vi "Version_4.9_8_on-chip_valves_for25ulSyringe_withModfied_Plunging.vi"() -> ()   [LabVIEW 2020] (continued)
                            n6063 = local write "Volume being Injected \nin this process"(0.0 ("Volume being Injected \nin this process")) -> ()
                          }
                        }
                      }
                      frame #5 {
                        n6064 = while {
                          stop <- w6523 stop-if-true
                          # "Re-introduce Sample into Column-2, Elute column-2 and Divert the sample onto Grid"
                          n6065 = local read "Start the Process"() -> (w6522:bool)
                          n6066 = case shown="True" w6522 {
                            frame False {
                            }
                            frame True {
                              n6067 = stacked-sequence {
                                frame #0 {
                                # "Reinitialize the pump"
                                n6068 = local read "VISA Refnum in\nfor Pump"() -> (w6525:refnum<visa-resource-name>)
                                n6069 = call "Initializer (SubVI).vi"("VISA Refnum in"=w6525) -> ()  [unwired: 11 in]
                                n6070 = local write "Re-SEC"(FALSE ("Re-SEC")) -> ()
                                }
                                frame #1 {
                                # "If Yes, this code will clean the column-2 with buffer-C prior to re-introducing the sample"
                                n6071 = local read "Wash column-2 Prior \nto re-introducing \nsample"() -> (w6526:bool)
                                n6072 = case shown="True" w6526 {
                                frame False {
                                }
                                frame True {
                                n6073 = stacked-sequence {
                                frame #0 {
                                n6074 = local read "VISA Refnum in\nfor Pump"() -> (w6528:refnum<visa-resource-name>)
                                n6075 = local read "Port for \nC2-Elution"() -> (w6527:string)
                                n6076 = call "PortChanger (SubVI).vi"("Port Number"=w6527, "VISA Refnum in"=w6528) -> ()  [unwired: 10 in]
                                }
                                frame #1 {
                                n6077 = local read "Stopper that ends \nthe main loops"() -> (w6529:bool)
                                n6078 = local read "VISA Refnum in\nfor Pump"() -> (w6530:refnum<visa-resource-name>)
                                n6079 = case shown="True" w6529 {
                                frame False {
                                }
                                frame True {
                                n6080 = local read "VISA Refnum in\nfor Pump"() -> (w6531:refnum<visa-resource-name>)
                                n6081 = call "HardStopCurrentProcess (SubVI).vi"("VISA Refnum in"=w6531) -> ()  [unwired: 11 in]
                                }
                                }
                                n6082 = call "ProcessCompletionWaiter (SubVI).vi"("VISA Refnum in"=w6530) -> ()  [unwired: 11 in]
                                }
                                frame #2 {
                                n6083 = local read "Buffer-B Pumping\nResolution"() -> (w6534:T2)
                                n6084 = local read "VISA Refnum in\nfor Pump"() -> (w6536:refnum<visa-resource-name>)
                                n6085 = local read "Buffer-C2 \nWash Volume\nPrior to re-introducing \nSample"() -> (w6533:dbl)
                                n6086 = local read "Volume of Syringe"() -> (w6535:dbl)
                                n6087 = call "RPickUp(SubVI).vi"("Volume to be picked up"=w6533, "Volume of Syringe"=w6535, "Resolution of PickUP"=w6534, "PickUp Flow Rate (ul/min)"=150.0, "VISA Refnum in"=w6536) -> ()  [unwired: 6 in, 1 out]
                                }
                                frame #3 {
                                n6088 = local read "Stopper that ends \nthe main loops"() -> (w6537:bool)
                                n6089 = local read "VISA Refnum in\nfor Pump"() -> (w6538:refnum<visa-resource-name>)
                                n6090 = case shown="True" w6537 {
                                frame False {
                                }
                                frame True {
                                n6091 = local read "VISA Refnum in\nfor Pump"() -> (w6539:refnum<visa-resource-name>)
                                n6092 = call "HardStopCurrentProcess (SubVI).vi"("VISA Refnum in"=w6539) -> ()  [unwired: 11 in]
                                }
                                }
                                n6093 = call "ProcessCompletionWaiter (SubVI).vi"("VISA Refnum in"=w6538) -> ()  [unwired: 11 in]
                                }
                                frame #4 {
                                n6094 = local read "VISA Refnum in\nfor Pump"() -> (w6541:refnum<visa-resource-name>)
                                n6095 = call "PortChanger (SubVI).vi"("Port Number"="10", "VISA Refnum in"=w6541) -> ()  [unwired: 10 in]
                                }
                                frame #5 {
                                n6096 = local read "Stopper that ends \nthe main loops"() -> (w6542:bool)
                                n6097 = local read "VISA Refnum in\nfor Pump"() -> (w6543:refnum<visa-resource-name>)
                                n6098 = case shown="True" w6542 {
                                frame False {
                                }
                                frame True {
                                n6099 = local read "VISA Refnum in\nfor Pump"() -> (w6544:refnum<visa-resource-name>)
                                n6100 = call "HardStopCurrentProcess (SubVI).vi"("VISA Refnum in"=w6544) -> ()  [unwired: 11 in]
                                }
                                }
                                n6101 = call "ProcessCompletionWaiter (SubVI).vi"("VISA Refnum in"=w6543) -> ()  [unwired: 11 in]
                                }
                                frame #6 {
                                n6102 = local read "Buffer-C2 Dispense \nFlow Rate for Washing \nPrior to re-introducing Sample"() -> (w6545:dbl)
                                n6103 = local read "VISA Refnum in\nfor Pump"() -> (w6549:refnum<visa-resource-name>)
                                n6104 = local read "Volume of Syringe"() -> (w6547:dbl)
                                n6105 = call "GoToAbsolutePosition(SubVI).vi"("Absolute Volume Position in Syringe (in ul)"=0.0, "Volume of Syringe"=w6547, "Resolution of Pumping"=T2."Standard Pumping", "Flow Rate (ul/min)"=w6545, "VISA Refnum in"=w6549) -> ()  [unwired: 6 in, 1 out]
                                }
                                frame #7 {
                                n6106 = local read "Stopper that ends \nthe main loops"() -> (w6550:bool)
                                n6107 = local read "VISA Refnum in\nfor Pump"() -> (w6551:refnum<visa-resource-name>)
                                n6108 = case shown="True" w6550 {
                                frame False {
                                }
                                frame True {
                                n6109 = local read "VISA Refnum in\nfor Pump"() -> (w6552:refnum<visa-resource-name>)
                                n6110 = call "HardStopCurrentProcess (SubVI).vi"("VISA Refnum in"=w6552) -> ()  [unwired: 11 in]
                                }
                                }
                                n6111 = call "ProcessCompletionWaiter (SubVI).vi"("VISA Refnum in"=w6551) -> ()  [unwired: 11 in]
                                }
                                }
                                }
                                }
                                }
                                frame #2 {
                                # "Switch to Port-7"
                                # "Port-7 of pump is connected to Buffer-B"
                                n6112 = local write "Washing Column-2"(FALSE ("Washing Column-2")) -> ()
                                n6113 = local read "VISA Refnum in\nfor Pump"() -> (w6559:refnum<visa-resource-name>)
                                n6114 = local read "Port for \nB-Elution"() -> (w6557:string)
                                n6115 = local write "Affinity Elution On"(TRUE ("Affinity Elution On")) -> ()
                                n6116 = call "PortChanger (SubVI).vi"("Port Number"=w6557, "VISA Refnum in"=w6559) -> ()  [unwired: 10 in]
                                n6117 = local write "Elution of Column-1"(TRUE ("Elution of Column-1")) -> ()
                                n6118 = local write "Clean the \nBuffer-B tubing"(FALSE ("Clean the \nBuffer-B tubing")) -> ()
                                n6119 = local write "Divert Sample \ninto Column-2"(TRUE ("Divert Sample \ninto Column-2")) -> ()
                                }
                                frame #3 {
                                n6120 = local read "VISA Refnum in\nfor Pump"() -> (w6560:refnum<visa-resource-name>)
                                n6121 = call "ProcessCompletionWaiter (SubVI).vi"("VISA Refnum in"=w6560) -> ()  [unwired: 11 in]
                                }
                                frame #4 {
                                # "If Yes, it will clean the elution buffer from port-5 tubing a bit more"
                                n6122 = local read "Clean the \nBuffer-B tubing"() -> (w6561:bool)
                                n6123 = case shown="True" w6561 {
                                frame False {
                                n6124 = stacked-sequence {
                                frame #0 {
                                n6125 = local read "Buffer-B Pumping\nResolution"() -> (w6564:T2)
                                n6126 = local read "VISA Refnum in\nfor Pump"() -> (w6566:refnum<visa-resource-name>)
                                n6127 = local read "V-S"() -> (w6563:dbl)
                                n6128 = local read "Volume of Syringe"() -> (w6565:dbl)
                                n6129 = call "RPickUp(SubVI).vi"("Volume to be picked up"=w6563, "Volume of Syringe"=w6565, "Resolution of PickUP"=w6564, "PickUp Flow Rate (ul/min)"=150.0, "VISA Refnum in"=w6566) -> ()  [unwired: 6 in, 1 out]
                                }
                                frame #1 {
                                n6130 = local read "Stopper that ends \nthe main loops"() -> (w6567:bool)
                                n6131 = local read "VISA Refnum in\nfor Pump"() -> (w6568:refnum<visa-resource-name>)
                                n6132 = case shown="True" w6567 {
                                frame False {
                                }
                                frame True {
                                n6133 = local read "VISA Refnum in\nfor Pump"() -> (w6569:refnum<visa-resource-name>)
                                n6134 = call "HardStopCurrentProcess (SubVI).vi"("VISA Refnum in"=w6569) -> ()  [unwired: 11 in]
                                }
                                }
                                n6135 = call "ProcessCompletionWaiter (SubVI).vi"("VISA Refnum in"=w6568) -> ()  [unwired: 11 in]
                                }
                                frame #2 {
                                n6136 = local read "VISA Refnum in\nfor Pump"() -> (w6571:refnum<visa-resource-name>)
                                n6137 = call "PortChanger (SubVI).vi"("Port Number"="1", "VISA Refnum in"=w6571) -> ()  [unwired: 10 in]
                                }
                                frame #3 {
                                n6138 = local read "Stopper that ends \nthe main loops"() -> (w6572:bool)
                                n6139 = local read "VISA Refnum in\nfor Pump"() -> (w6573:refnum<visa-resource-name>)
                                n6140 = case shown="True" w6572 {
                                frame False {
                                }
                                frame True {
                                n6141 = local read "VISA Refnum in\nfor Pump"() -> (w6574:refnum<visa-resource-name>)
                                n6142 = call "HardStopCurrentProcess (SubVI).vi"("VISA Refnum in"=w6574) -> ()  [unwired: 11 in]
                                }
                                }
                                n6143 = call "ProcessCompletionWaiter (SubVI).vi"("VISA Refnum in"=w6573) -> ()  [unwired: 11 in]
                                }
                                frame #4 {
                                n6144 = local read "VISA Refnum in\nfor Pump"() -> (w6579:refnum<visa-resource-name>)
                                n6145 = local read "Volume of Syringe"() -> (w6576:dbl)
                                n6146 = call "GoToAbsolutePosition(SubVI).vi"("Absolute Volume Position in Syringe (in ul)"=0.0, "Volume of Syringe"=w6576, "Resolution of Pumping"=T2."Standard Pumping", "Flow Rate (ul/min)"=150.0, "VISA Refnum in"=w6579) -> ()  [unwired: 6 in, 1 out]
                                }
                                frame #5 {
                                n6147 = local read "Stopper that ends \nthe main loops"() -> (w6580:bool)
                                n6148 = local read "VISA Refnum in\nfor Pump"() -> (w6581:refnum<visa-resource-name>)
                                n6149 = case shown="True" w6580 {
                                frame False {
                                }
                                frame True {
                                n6150 = local read "VISA Refnum in\nfor Pump"() -> (w6582:refnum<visa-resource-name>)
                                n6151 = call "HardStopCurrentProcess (SubVI).vi"("VISA Refnum in"=w6582) -> ()  [unwired: 11 in]
                                }
                                }
                                n6152 = call "ProcessCompletionWaiter (SubVI).vi"("VISA Refnum in"=w6581) -> ()  [unwired: 11 in]
                                }
                                }
                                }
                                frame True {
                                n6153 = for {
                                N: 2 -> [_]
                                n6154 = stacked-sequence {
                                frame #0 {
                                n6155 = local read "Buffer-B Pumping\nResolution"() -> (w6586:T2)
                                n6156 = local read "VISA Refnum in\nfor Pump"() -> (w6588:refnum<visa-resource-name>)
                                n6157 = local read "Apparent Volume\nof Syringe"() -> (w6585:dbl)
                                n6158 = local read "Volume of Syringe"() -> (w6587:dbl)
                                n6159 = call "RPickUp(SubVI).vi"("Volume to be picked up"=w6585, "Volume of Syringe"=w6587, "Resolution of PickUP"=w6586, "PickUp Flow Rate (ul/min)"=150.0, "VISA Refnum in"=w6588) -> ()  [unwired: 6 in, 1 out]
                                }
                                frame #1 {
                                n6160 = local read "Stopper that ends \nthe main loops"() -> (w6589:bool)
                                n6161 = local read "VISA Refnum in\nfor Pump"() -> (w6590:refnum<visa-resource-name>)
                                n6162 = case shown="True" w6589 {
                                frame False {
                                }
                                frame True {
                                n6163 = local read "VISA Refnum in\nfor Pump"() -> (w6591:refnum<visa-resource-name>)
                                n6164 = call "HardStopCurrentProcess (SubVI).vi"("VISA Refnum in"=w6591) -> ()  [unwired: 11 in]
                                }
                                }
                                n6165 = call "ProcessCompletionWaiter (SubVI).vi"("VISA Refnum in"=w6590) -> ()  [unwired: 11 in]
                                }
                                frame #2 {
                                n6166 = local read "VISA Refnum in\nfor Pump"() -> (w6593:refnum<visa-resource-name>)
                                n6167 = call "PortChanger (SubVI).vi"("Port Number"="1", "VISA Refnum in"=w6593) -> ()  [unwired: 10 in]
                                }
                                frame #3 {
                                n6168 = local read "Stopper that ends \nthe main loops"() -> (w6594:bool)
                                n6169 = local read "VISA Refnum in\nfor Pump"() -> (w6595:refnum<visa-resource-name>)
                                n6170 = case shown="True" w6594 {
                                frame False {
                                }
                                frame True {
                                n6171 = local read "VISA Refnum in\nfor Pump"() -> (w6596:refnum<visa-resource-name>)
                                n6172 = call "HardStopCurrentProcess (SubVI).vi"("VISA Refnum in"=w6596) -> ()  [unwired: 11 in]
                                }
                                }
                                n6173 = call "ProcessCompletionWaiter (SubVI).vi"("VISA Refnum in"=w6595) -> ()  [unwired: 11 in]
                                }
                                frame #4 {
                                n6174 = local read "VISA Refnum in\nfor Pump"() -> (w6601:refnum<visa-resource-name>)
                                n6175 = local read "Volume of Syringe"() -> (w6598:dbl)
                                n6176 = call "GoToAbsolutePosition(SubVI).vi"("Absolute Volume Position in Syringe (in ul)"=0.0, "Volume of Syringe"=w6598, "Resolution of Pumping"=T2."Standard Pumping", "Flow Rate (ul/min)"=150.0, "VISA Refnum in"=w6601) -> ()  [unwired: 6 in, 1 out]
                                }
                                frame #5 {
                                n6177 = local read "Stopper that ends \nthe main loops"() -> (w6602:bool)
                                n6178 = local read "VISA Refnum in\nfor Pump"() -> (w6603:refnum<visa-resource-name>)
                                n6179 = case shown="True" w6602 {
                                frame False {
                                }
                                frame True {
                                n6180 = local read "VISA Refnum in\nfor Pump"() -> (w6604:refnum<visa-resource-name>)
                                n6181 = call "HardStopCurrentProcess (SubVI).vi"("VISA Refnum in"=w6604) -> ()  [unwired: 11 in]
                                }
                                }
                                n6182 = call "ProcessCompletionWaiter (SubVI).vi"("VISA Refnum in"=w6603) -> ()  [unwired: 11 in]
                                }
                                }
                                }
                                }
                                }
                                }
                                frame #5 {
                                n6183 = local read "VISA Refnum in\nfor Pump"() -> (w6606:refnum<visa-resource-name>)
                                n6184 = local read "Port for \nB-Elution"() -> (w6605:string)
                                n6185 = call "PortChanger (SubVI).vi"("Port Number"=w6605, "VISA Refnum in"=w6606) -> ()  [unwired: 10 in]
                                }
                                frame #6 {
                                n6186 = local read "VISA Refnum in\nfor Pump"() -> (w6607:refnum<visa-resource-name>)
                                n6187 = call "ProcessCompletionWaiter (SubVI).vi"("VISA Refnum in"=w6607) -> ()  [unwired: 11 in]
                                }
                                frame #7 {
                                n6188 = local read "Buffer-B PickUp \nFlow Rate (ul/min)"() -> (w6610:dbl)
                                n6189 = local read "Buffer-B Pumping\nResolution"() -> (w6609:T2)
                                n6190 = local read "VISA Refnum in\nfor Pump"() -> (w6612:refnum<visa-resource-name>)
                                n6191 = local read "Buffer-B Volume \nto be  Pumped"() -> (w6608:dbl)
                                n6192 = local read "Volume of Syringe"() -> (w6611:dbl)
                                n6193 = call "RPickUp(SubVI).vi"("Volume to be picked up"=w6608, "Volume of Syringe"=w6611, "Resolution of PickUP"=w6609, "PickUp Flow Rate (ul/min)"=w6610, "VISA Refnum in"=w6612) -> ()  [unwired: 6 in, 1 out]
                                }
                                frame #8 {
                                n6194 = local read "Stopper that ends \nthe main loops"() -> (w6613:bool)
                                n6195 = local read "VISA Refnum in\nfor Pump"() -> (w6614:refnum<visa-resource-name>)
                                n6196 = case shown="True" w6613 {
                                frame False {
                                }
                                frame True {
                                n6197 = local read "VISA Refnum in\nfor Pump"() -> (w6615:refnum<visa-resource-name>)
                                n6198 = call "HardStopCurrentProcess (SubVI).vi"("VISA Refnum in"=w6615) -> ()  [unwired: 11 in]
                                }
                                }
                                n6199 = call "ProcessCompletionWaiter (SubVI).vi"("VISA Refnum in"=w6614) -> ()  [unwired: 11 in]
                                }
                                frame #9 {
                                # "Reads the initial Plunger Position for computing the volume dispensed"
                                n6200 = local read "VISA Refnum in\nfor Pump"() -> (w6617:refnum<visa-resource-name>)
                                n6201 = call "AbsolutePlungerPosition (SubVI).vi"("VISA Refnum in"=w6617) -> ("Plunger Position"=w6616:i32)  [unwired: 10 in]
                                n6202 = local write "Initial Plunger Position"(w6616) -> ()
                                }
                                frame #10 {
                                # "Switch to Port-2"
                                # "Port-2 of the pump is conncted to column-1 of chip"
                                n6203 = local read "VISA Refnum in\nfor Pump"() -> (w6619:refnum<visa-resource-name>)
                                n6204 = call "PortChanger (SubVI).vi"("Port Number"="2", "VISA Refnum in"=w6619) -> ()  [unwired: 10 in]
                                }
                                frame #11 {
                                n6205 = local read "Stopper that ends \nthe main loops"() -> (w6620:bool)
                                n6206 = local read "VISA Refnum in\nfor Pump"() -> (w6621:refnum<visa-resource-name>)
                                n6207 = call "ProcessCompletionWaiter (SubVI).vi"("VISA Refnum in"=w6621) -> ()  [unwired: 11 in]
                                n6208 = case shown="True" w6620 {
                                frame False {
                                }
                                frame True {
                                n6209 = local read "VISA Refnum in\nfor Pump"() -> (w6622:refnum<visa-resource-name>)
                                n6210 = call "HardStopCurrentProcess (SubVI).vi"("VISA Refnum in"=w6622) -> ()  [unwired: 11 in]
                                }
                                }
                                }
                                frame #12 {
                                # "Keeps the AMF valve after column-1 open and valve after column-2 closed"
                                n6211 = local read "VISA Refnum in\nfor Valve"() -> (w6627:refnum<visa-resource-name>)
                                n6212 = local read "External Valve \nOPEN"() -> (w6626:string)
                                n6213 = call "PortChanger_Valve (SubVI).vi"("Port Number"=w6626, "VISA Refnum in"=w6627) -> ()  [unwired: 10 in]
                                n6214 = local write "Valve V1 Open"(TRUE ("Valve V1 Open")) -> ()
                                n6215 = local write "Valve V2 Open"(TRUE ("Valve V2 Open")) -> ()
                                n6216 = local write "Valve V3 Open"(FALSE ("Valve V3 Open")) -> ()
                                n6217 = local write "Valve V4 Open"(FALSE ("Valve V4 Open")) -> ()
                                n6218 = local write "Valve V6 Open"(FALSE ("Valve V6 Open")) -> ()
                                n6219 = local write "Valve V5 Open"(FALSE ("Valve V5 Open")) -> ()
                                n6220 = local write "Valve V7 Open"(FALSE ("Valve V7 Open")) -> ()
                                }
                                frame #13 {
                                n6221 = local read "Buffer-B Dispense\nFlow Rate (ul/min)"() -> (w6637:dbl)
                                n6222 = local read "Buffer-B Pumping\nResolution"() -> (w6636:T2)
                                n6223 = local read "Initial Plunger Position"() -> (w6633:dbl)
                                n6224 = local read "VISA Refnum in\nfor Pump"() -> (w6639:refnum<visa-resource-name>)
                                n6225 = local read "Volume of Syringe"() -> (w6638:dbl)
                                n6226 = call "GoToAbsolutePosition(SubVI).vi"("Absolute Volume Position in Syringe (in ul)"=0.0 ("Volume to be Dispensed"), "Volume of Syringe"=w6638, "Resolution of Pumping"=w6636, "Flow Rate (ul/min)"=w6637, "VISA Refnum in"=w6639) -> ()  [unwired: 6 in, 1 out]
                                n6227 = local write "Pause Data Collection"(FALSE ("Pause Data Collection")) -> ()
                                n6228 = local write "Vol_now"(0.0 ("Vol_now")) -> ()
                                n6229 = local write "Position\nNow"(w6633) -> ()
                                }
                                frame #14 {
                                n6230 = while {
                                stop <- w6646 stop-if-true
                                n6231 = event shown="[0] \"Pause Elution Value\": Value Change" {
                                selector: _ -> [_ _]
                                dyn-events: _ -> [_ _]
                                timeout: 100 -> [_ _]
                                event "Pause Elution\nValue": Value Change {
                                n6232 = event-data() -> ()  [unwired: 1 in, 6 out]
                                n6233 = stacked-sequence {
                                frame #0 {
                                n6234 = local read "Pause Elution"() -> (w6648:bool)
                                n6235 = case shown="False" w6648 {
                                frame False {
                                n6236 = local write "Pause Elution"(TRUE ("Pause Elution")) -> ()
                                }
                                frame True {
                                n6237 = local write "Pause Elution"(FALSE ("Pause Elution")) -> ()
                                }
                                }
                                }
                                frame #1 {
                                n6238 = local read "Pause Elution"() -> (w6651:bool)
                                n6239 = case shown="False" w6651 {
                                frame False {
                                n6240 = local read "Buffer-B Dispense\nFlow Rate (ul/min)"() -> (w6656:dbl)
                                n6241 = local read "VISA Refnum in\nfor Pump"() -> (w6657:refnum<visa-resource-name>)
                                n6242 = local read "Buffer-B Pumping\nResolution"() -> (w6653:T2)
                                n6243 = local read "Volume of Syringe"() -> (w6654:dbl)
                                n6244 = call "GoToAbsolutePosition(SubVI).vi"("Absolute Volume Position in Syringe (in ul)"=0.0, "Volume of Syringe"=w6654, "Resolution of Pumping"=w6653, "Flow Rate (ul/min)"=w6656, "VISA Refnum in"=w6657) -> ()  [unwired: 6 in, 1 out]
                                n6245 = local write "Pause Data Collection"(FALSE ("Pause Data Collection")) -> ()
                                }
                                frame True {
                                n6246 = local read "VISA Refnum in\nfor Pump"() -> (w6659:refnum<visa-resource-name>)
                                n6247 = local write "Pause Data Collection"(TRUE ("Pause Data Collection")) -> ()
                                n6248 = call "HardStopCurrentProcess (SubVI).vi"("VISA Refnum in"=w6659) -> ()  [unwired: 11 in]
                                }
                                }
                                }
                                }
                                }
                                event Timeout {
                                n6249 = event-data() -> ()  [unwired: 1 in, 3 out]
                                }
                                }
                                n6250 = local read "Divert Sample \ninto Column-2"() -> (w6644:bool)
                                n6251 = local read "Stopper that ends \nthe main loops"() -> (w6645:bool)
                                n6252 = Or(x=w6644, y=w6645) -> (x .or. y?=w6646:bool)
                                }
                                n6253 = local read "Buffer-B Pumping\nResolution"() -> (w6642:T2)
                                n6254 = local read "VISA Refnum in\nfor Pump"() -> (w6643:refnum<visa-resource-name>)
                                n6255 = local read "Volume of Syringe"() -> (w6641:dbl)
                                n6256 = while {
                                tunnel: w6643 -> [w6668]
                                tunnel: w6642 -> [w6667]
                                tunnel: w6641 -> [w6666]
                                stop <- w6662 stop-if-true
                                n6257 = local read "Position\nNow"() -> (w6660:dbl)
                                n6258 = local read "Pause Elution"() -> (w6661:bool)
                                n6259 = case shown="True" w6661 {
                                tunnel: w6660 -> [w6672 _]
                                tunnel: w6668 -> [w6671 w6714]
                                tunnel: w6667 -> [w6670 _]
                                tunnel: w6666 -> [w6669 _]
                                frame False {
                                n6260 = stacked-sequence {
                                tunnel: w6672 -> [_ w6678]
                                tunnel: w6671 -> [_ w6677]
                                tunnel: w6670 -> [_ w6676]
                                tunnel: w6669 -> [_ w6675]
                                frame #0 {
                                n6261 = Wait (ms)(milliseconds to wait=u32 3000) -> ()  [unwired: 1 out]
                                n6262 = local write "Signal"(TRUE ("Signal")) -> ()
                                }
                                frame #1 {
                                n6263 = while {
                                tunnel: w6678 -> [w6690]
                                tunnel: w6677 -> [w6689]
                                tunnel: w6676 -> [w6688]
                                tunnel: w6675 -> [w6687]
                                stop <- w6682 stop-if-true
                                n6264 = stacked-sequence {
                                tunnel: w6690 -> [_ w6697]
                                tunnel: w6689 -> [_ w6696]
                                tunnel: w6688 -> [_ w6695]
                                tunnel: w6687 -> [_ w6694]
                                frame #0 {
                                n6265 = Wait (ms)(milliseconds to wait=u32 500) -> ()  [unwired: 1 out]
                                }
                                frame #1 {
                                n6266 = call "AbsolutePlungerPosition (SubVI).vi"("VISA Refnum in"=w6696) -> ("Plunger Position"=w6693:i32)  [unwired: 10 in]
                                n6267 = case shown="\"High Resolution Pumping\"" w6695 {
                                tunnel: w6697 -> [w6702 w6711]
                                tunnel: w6693 -> [w6703 w6710]
                                tunnel: [w6701 w6708] -> w6692
                                tunnel: w6694 -> [w6700 w6709]
                                frame "Standard Pumping", Default {
                                n6268 = Subtract(x=w6702, y=w6703) -> (x-y=w6699:dbl)
                                n6269 = Absolute Value(x=w6699) -> (abs(x)=w6698:dbl)
                                n6270 = Multiply(x=w6698, y=w6700) -> (x*y=w6705:dbl)
                                n6271 = Divide(x=w6705, y=3000.0) -> (x/y=w6701:dbl)
                                }
                                frame "High Resolution Pumping" {
                                n6272 = Subtract(x=w6711, y=w6710) -> (x-y=w6707:dbl)
                                n6273 = Absolute Value(x=w6707) -> (abs(x)=w6706:dbl)
                                n6274 = Multiply(x=w6706, y=w6709) -> (x*y=w6713:dbl)
                                n6275 = Divide(x=w6713, y=24000.0) -> (x/y=w6708:dbl)
                                }
                                }
                                n6276 = local write "Volume being Injected \nin this process"(w6692) -> ()
                                }
                                }
                                n6277 = local read "Volume being Injected \nin this process"() -> (w6680:dbl)
                                n6278 = local read "Affinity Elution \nGraph Min CutOff"() -> (w6679:dbl)
                                n6279 = local read "Stopper that ends \nthe main loops"() -> (w6685:bool)
                                n6280 = local read "Divert Sample \ninto Column-2"() -> (w6686:bool)
                                n6281 = Greater Or Equal?(x=w6680, y=w6679) -> (x >= y?=w6681:bool)
                                n6282 = Or(x=w6686, y=w6685) -> (x .or. y?=w6683:bool)
                                n6283 = local read "Pause Elution"() -> (w6684:bool)
                                n6284 = local write "Affinity Elution \nis Approaching"(w6681) -> ()
                                n6285 = Or(x=w6684, y=w6683) -> (x .or. y?=w6682:bool)
                                }
                                }
                                }
                                }
                                frame True {
                                n6286 = stacked-sequence {
                                tunnel: w6714 -> [_ w6717 _]
                                frame #0 {
                                n6287 = Wait (ms)(milliseconds to wait=u32 2000) -> ()  [unwired: 1 out]
                                }
                                frame #1 {
                                n6288 = local read "Signal"() -> (w6716:bool)
                                n6289 = case shown="True" w6716 {
                                tunnel: w6717 -> [_ w6723]
                                frame False {
                                }
                                frame True {
                                n6290 = local read "Volume being Injected \nin this process"() -> (w6721:dbl)
                                n6291 = local read "Net Elution \nVolume"() -> (w6720:dbl)
                                n6292 = local write "Signal"(FALSE ("Signal")) -> ()
                                n6293 = Add(x=w6721, y=w6720) -> (x+y=w6719:dbl)
                                n6294 = call "AbsolutePlungerPosition (SubVI).vi"("VISA Refnum in"=w6723) -> ("Plunger Position"=w6722:i32)  [unwired: 10 in]
                                n6295 = local write "Net Elution \nVolume"(w6719) -> ()
                                n6296 = local write "Position\nNow"(w6722) -> ()
                                }
                                }
                                }
                                frame #2 {
                                n6297 = local write "Volume being Injected \nin this process"(0.0 ("Volume being Injected \nin this process")) -> ()
                                }
                                }
                                }
                                }
                                n6298 = local read "Stopper that ends \nthe main loops"() -> (w6664:bool)
                                n6299 = local read "Divert Sample \ninto Column-2"() -> (w6663:bool)
                                n6300 = Or(x=w6663, y=w6664) -> (x .or. y?=w6662:bool)
                                n6301 = Wait (ms)(milliseconds to wait=u32 300) -> ()  [unwired: 1 out]
                                }
                                n6302 = local read "Stopper that ends \nthe main loops"() -> (w6640:bool)
                                n6303 = case shown="True" w6640 {
                                frame False {
                                }
                                frame True {
                                n6304 = local read "VISA Refnum in\nfor Pump"() -> (w6725:refnum<visa-resource-name>)
                                n6305 = call "HardStopCurrentProcess (SubVI).vi"("VISA Refnum in"=w6725) -> ()  [unwired: 11 in]
                                }
                                }
                                }
                                frame #15 {
                                # "valve after column-1 is closed"
                                # "Keeps the on-chip Valve V1 and V3 after column-2 open"
                                # "Keeps the AMF valve after column-1 closed and valve after column-2 open"
                                n6306 = local read "VISA Refnum in\nfor Pump"() -> (w6738:refnum<visa-resource-name>)
                                n6307 = local read "Volume being Injected \nin this process"() -> (w6735:dbl)
                                n6308 = local write "Sample Volume Diverted\ninto Column-2"(0.0 ("Sample Volume Diverted\ninto Column-2")) -> ()
                                n6309 = call "AbsolutePlungerPosition (SubVI).vi"("VISA Refnum in"=w6738) -> ("Plunger Position"=w6737:i32)  [unwired: 10 in]
                                n6310 = local write "Position\nNow"(w6737) -> ()
                                n6311 = local write "Vol_previous"(0.0 ("Vol_diff")) -> ()
                                n6312 = local write "Vol_now"(w6735) -> ()
                                n6313 = local read "VISA Refnum in\nfor Valve"() -> (w6730:refnum<visa-resource-name>)
                                n6314 = local read "External Valve \nCLOSED"() -> (w6729:string)
                                n6315 = local write "Valve V1 Open"(TRUE ("Valve V1 Open")) -> ()
                                n6316 = local write "Valve V3 Open"(TRUE ("Valve V3 Open")) -> ()
                                n6317 = local write "Valve V2 Open"(FALSE ("Valve V2 Open")) -> ()
                                n6318 = local write "Valve V4 Open"(TRUE ("Valve V4 Open")) -> ()
                                n6319 = call "PortChanger_Valve (SubVI).vi"("Port Number"=w6729, "VISA Refnum in"=w6730) -> ()  [unwired: 10 in]
                                n6320 = local write "Valve V5 Open"(TRUE ("Valve V5 Open")) -> ()
                                n6321 = local write "Valve V6 Open"(FALSE ("Valve V6 Open")) -> ()
                                n6322 = local write "Valve V7 Open"(TRUE ("Valve V7 Open")) -> ()
                                }
                                frame #16 {
                                n6323 = local read "Divert Sample \ninto Column-2"() -> (w6740:bool)
                                n6324 = case shown="True" w6740 {
                                frame False {
                                n6325 = stacked-sequence {
                                frame #0 {
                                n6326 = local read "Buffer-B Pumping\nResolution"() -> (w6743:T2)
                                n6327 = local read "VISA Refnum in\nfor Pump"() -> (w6745:refnum<visa-resource-name>)
                                n6328 = local read "Initial Plunger Position"() -> (w6744:dbl)
                                n6329 = local read "Volume of Syringe"() -> (w6742:dbl)
                                n6330 = while {
                                tunnel: w6744 -> [w6751]
                                tunnel: w6745 -> [w6750]
                                tunnel: w6743 -> [w6749]
                                tunnel: w6742 -> [w6748]
                                stop <- w6746 stop-if-true
                                n6331 = Wait (ms)(milliseconds to wait=u32 100) -> ()  [unwired: 1 out]
                                n6332 = stacked-sequence {
                                tunnel: w6751 -> [w6757 _]
                                tunnel: w6750 -> [w6756 w6777]
                                tunnel: w6749 -> [w6755 _]
                                tunnel: w6748 -> [w6754 _]
                                tunnel: [_ w6775] -> w6746
                                frame #0 {
                                n6333 = call "AbsolutePlungerPosition (SubVI).vi"("VISA Refnum in"=w6756) -> ("Plunger Position"=w6753:i32)  [unwired: 10 in]
                                n6334 = case shown="\"Standard Pumping\", Default" w6755 {
                                tunnel: w6757 -> [w6762 w6771]
                                tunnel: w6753 -> [w6763 w6770]
                                tunnel: [w6761 w6768] -> w6752
                                tunnel: w6754 -> [w6760 w6769]
                                frame "Standard Pumping", Default {
                                n6335 = Subtract(x=w6762, y=w6763) -> (x-y=w6759:dbl)
                                n6336 = Absolute Value(x=w6759) -> (abs(x)=w6758:dbl)
                                n6337 = Multiply(x=w6758, y=w6760) -> (x*y=w6765:dbl)
                                n6338 = Divide(x=w6765, y=3000.0) -> (x/y=w6761:dbl)
                                }
                                frame "High Resolution Pumping" {
                                n6339 = Subtract(x=w6771, y=w6770) -> (x-y=w6767:dbl)
                                n6340 = Absolute Value(x=w6767) -> (abs(x)=w6766:dbl)
                                n6341 = Multiply(x=w6766, y=w6769) -> (x*y=w6773:dbl)
                                n6342 = Divide(x=w6773, y=24000.0) -> (x/y=w6768:dbl)
                                }
                                }
                                n6343 = local write "Volume being Injected \nin this process"(w6752) -> ()
                                }
                                frame #1 {
                                n6344 = local read "Stopper that ends \nthe main loops"() -> (w6774:bool)
                                n6345 = call "LSPOneStatus (SubVI).vi"("VISA Refnum in"=w6777) -> ("read buffer"=w6779:string)  [unwired: 10 in]
                                n6346 = call <vilib>:"Trim Whitespace.vi"("string"=w6779) -> ("trimmed string"=w6778:string)  [unwired: 1 in]
                                n6347 = Equal?(x=w6778, y="/0`\u0003") -> (x = y?=w6776:bool)
                                n6348 = Or(x=w6776, y=w6774) -> (x .or. y?=w6775:bool)
                                }
                                }
                                }
                                n6349 = local read "Stopper that ends \nthe main loops"() -> (w6741:bool)
                                n6350 = case shown="True" w6741 {
                                frame False {
                                }
                                frame True {
                                n6351 = local read "VISA Refnum in\nfor Pump"() -> (w6781:refnum<visa-resource-name>)
                                n6352 = call "HardStopCurrentProcess (SubVI).vi"("VISA Refnum in"=w6781) -> ()  [unwired: 11 in]
                                }
                                }
                                }
                                }
                                }
                                frame True {
                                n6353 = stacked-sequence {
                                frame #0 {
                                n6354 = local read "Buffer-B Pumping\nResolution"() -> (w6784:T2)
                                n6355 = local read "VISA Refnum in\nfor Pump"() -> (w6786:refnum<visa-resource-name>)
                                n6356 = local read "Volume of Syringe"() -> (w6783:dbl)
                                n6357 = local read "Position\nNow"() -> (w6785:dbl)
                                n6358 = while {
                                tunnel: w6785 -> [w6792]
                                tunnel: w6786 -> [w6791]
                                tunnel: w6784 -> [w6790]
                                tunnel: w6783 -> [w6789]
                                stop <- w6787 stop-if-true
                                n6359 = Wait (ms)(milliseconds to wait=u32 100) -> ()  [unwired: 1 out]
                                n6360 = stacked-sequence {
                                tunnel: w6792 -> [w6802 _ _]
                                tunnel: w6791 -> [w6801 _ w6828]
                                tunnel: w6790 -> [w6800 _ _]
                                tunnel: w6789 -> [w6799 _ _]
                                tunnel: [_ _ w6826] -> w6787
                                frame #0 {
                                n6361 = local read "Vol_previous"() -> (w6796:dbl)
                                n6362 = call "AbsolutePlungerPosition (SubVI).vi"("VISA Refnum in"=w6801) -> ("Plunger Position"=w6798:i32)  [unwired: 10 in]
                                n6363 = case shown="\"Standard Pumping\", Default" w6800 {
                                tunnel: w6802 -> [w6807 w6816]
                                tunnel: w6798 -> [w6808 w6815]
                                tunnel: [w6806 w6813] -> w6797
                                tunnel: w6799 -> [w6805 w6814]
                                frame "Standard Pumping", Default {
                                n6364 = Subtract(x=w6807, y=w6808) -> (x-y=w6804:dbl)
                                n6365 = Absolute Value(x=w6804) -> (abs(x)=w6803:dbl)
                                n6366 = Multiply(x=w6803, y=w6805) -> (x*y=w6810:dbl)
                                n6367 = Divide(x=w6810, y=3000.0) -> (x/y=w6806:dbl)
                                }
                                frame "High Resolution Pumping" {
                                n6368 = Subtract(x=w6816, y=w6815) -> (x-y=w6812:dbl)
                                n6369 = Absolute Value(x=w6812) -> (abs(x)=w6811:dbl)
                                n6370 = Multiply(x=w6811, y=w6814) -> (x*y=w6818:dbl)
                                n6371 = Divide(x=w6818, y=24000.0) -> (x/y=w6813:dbl)
                                }
                                }
                                n6372 = Subtract(x=w6797, y=w6796) -> (x-y=w6795:dbl)
                                n6373 = local read "Vol_now"() -> (w6793:dbl)
                                n6374 = local write "Sample Volume Diverted\ninto Column-2"(w6797) -> ()
                                n6375 = Add(x=w6795, y=w6793) -> (x+y=w6794:dbl)
                                n6376 = local write "Volume being Injected \nin this process"(w6794) -> ()
                                }
                                frame #1 {
                                n6377 = local read "Volume being Injected \nin this process"() -> (w6819:dbl)
                                n6378 = local read "Sample Volume Diverted\ninto Column-2"() -> (w6820:dbl)
                                n6379 = local write "Vol_now"(w6819) -> ()
                                n6380 = local write "Vol_previous"(w6820) -> ()
                                }
                                frame #2 {
                                n6381 = local read "Buffer-B Volume \nto be Pumped for\nSample Diversion\nto Column-2"() -> (w6822:dbl)
                                n6382 = local read "Sample Volume Diverted\ninto Column-2"() -> (w6821:dbl)
                                n6383 = local read "Stopper that ends \nthe main loops"() -> (w6823:bool)
                                n6384 = call "LSPOneStatus (SubVI).vi"("VISA Refnum in"=w6828) -> ("read buffer"=w6830:string)  [unwired: 10 in]
                                n6385 = call <vilib>:"Trim Whitespace.vi"("string"=w6830) -> ("trimmed string"=w6829:string)  [unwired: 1 in]
                                n6386 = Equal?(x=w6829, y="/0`\u0003") -> (x = y?=w6827:bool)
                                n6387 = Greater Or Equal?(x=w6821, y=w6822) -> (x >= y?=w6825:bool)
                                n6388 = Or(x=w6823, y=w6825) -> (x .or. y?=w6824:bool)
                                n6389 = Or(x=w6827, y=w6824) -> (x .or. y?=w6826:bool)
                                }
                                }
                                }
                                n6390 = local read "Stopper that ends \nthe main loops"() -> (w6782:bool)
                                n6391 = case shown="True" w6782 {
                                frame False {
                                }
                                frame True {
                                n6392 = local read "VISA Refnum in\nfor Pump"() -> (w6832:refnum<visa-resource-name>)
                                n6393 = call "HardStopCurrentProcess (SubVI).vi"("VISA Refnum in"=w6832) -> ()  [unwired: 11 in]
                                }
                                }
                                }
                                frame #1 {
                                n6394 = local read "VISA Refnum in\nfor Pump"() -> (w6834:refnum<visa-resource-name>)
                                n6395 = local write "Pause Data Collection"(TRUE ("Pause Data Collection")) -> ()
                                n6396 = call "HardStopCurrentProcess (SubVI).vi"("VISA Refnum in"=w6834) -> ()  [unwired: 11 in]
                                }
                                frame #2 {
                                n6397 = local read "VISA Refnum in\nfor Pump"() -> (w6835:refnum<visa-resource-name>)
                                n6398 = call "PortChanger (SubVI).vi"("Port Number"="1", "VISA Refnum in"=w6835) -> ()  [unwired: 10 in]
                                }
                                frame #3 {
                                n6399 = local read "VISA Refnum in\nfor Pump"() -> (w6841:refnum<visa-resource-name>)
                                n6400 = local read "Volume of Syringe"() -> (w6837:dbl)
                                n6401 = call "GoToAbsolutePosition(SubVI).vi"("Absolute Volume Position in Syringe (in ul)"=0.0, "Volume of Syringe"=w6837, "Resolution of Pumping"=T2."Standard Pumping", "Flow Rate (ul/min)"=150.0, "VISA Refnum in"=w6841) -> ()  [unwired: 6 in, 1 out]
                                }
                                frame #4 {
                                n6402 = local read "VISA Refnum in\nfor Pump"() -> (w6843:refnum<visa-resource-name>)
                                n6403 = local write "Divert Sample \ninto Column-2"(FALSE ("Divert Sample \ninto Column-2")) -> ()
                                n6404 = call "ProcessCompletionWaiter (SubVI).vi"("VISA Refnum in"=w6843) -> ()  [unwired: 11 in]
                                }
                                }
                                }
                                }
                                }
                                frame #17 {
                                # "Keeps the On-Chip Valves V1 and V3 closed"
                                # "Switch to Port-5/8"
                                # "Port-5/8 of pump is connected to Buffer-C1/C2"
                                # "Keeps the AMF valve after column-1 open and valve after column-2 closed"
                                n6405 = local read "VISA Refnum in\nfor Pump"() -> (w6856:refnum<visa-resource-name>)
                                n6406 = local write "Pause Data Collection"(TRUE ("Pause Data Collection")) -> ()
                                n6407 = Wait (ms)(milliseconds to wait=u32 500) -> ()  [unwired: 1 out]
                                n6408 = local write "Affinity On"(FALSE ("Affinity On")) -> ()
                                n6409 = local read "Port for \nC2-Elution"() -> (w6847:string)
                                n6410 = local write "Affinity Elution On"(FALSE ("Affinity Elution On")) -> ()
                                n6411 = call "PortChanger (SubVI).vi"("Port Number"=w6847, "VISA Refnum in"=w6856) -> ()  [unwired: 10 in]
                                n6412 = local read "VISA Refnum in\nfor Valve"() -> (w6850:refnum<visa-resource-name>)
                                n6413 = local read "External Valve \nCLOSED"() -> (w6849:string)
                                n6414 = local write "Valve V1 Open"(FALSE ("Valve V1 Open")) -> ()
                                n6415 = local write "Valve V2 Open"(FALSE ("Valve V2 Open")) -> ()
                                n6416 = local write "Valve V3 Open"(FALSE ("Valve V3 Open")) -> ()
                                n6417 = local write "Valve V4 Open"(FALSE ("Valve V4 Open")) -> ()
                                n6418 = call "PortChanger_Valve (SubVI).vi"("Port Number"=w6849, "VISA Refnum in"=w6850) -> ()  [unwired: 10 in]
                                n6419 = local write "Valve V5 Open"(FALSE ("Valve V5 Open")) -> ()
                                n6420 = local write "Valve V6 Open"(FALSE ("Valve V6 Open")) -> ()
                                n6421 = local write "Valve V7 Open"(FALSE ("Valve V7 Open")) -> ()
                                }
                                frame #18 {
                                n6422 = local read "VISA Refnum in\nfor Pump"() -> (w6860:refnum<visa-resource-name>)
                                n6423 = call "ProcessCompletionWaiter (SubVI).vi"("VISA Refnum in"=w6860) -> ()  [unwired: 11 in]
                                n6424 = local write "Start the Process"(FALSE ("Start the Process")) -> ()
                                }
                                frame #19 {
                                n6425 = local read "Stopper that ends \nthe main loops"() -> (w6864:bool)
                                n6426 = local read "Start the Process"() -> (w6865:bool)
                                n6427 = Or(x=w6865, y=w6864) -> (x .or. y?=w6863:bool)
                                n6428 = local write "Elution of Column-1"(FALSE ("Elution of Column-1")) -> ()
                                n6429 = case shown="False" w6863 {
                                frame False {
                                n6430 = while {
                                stop <- w6869 stop-if-true
                                n6431 = local read "Stopper that ends \nthe main loops"() -> (w6870:bool)
                                n6432 = local read "Start the Process"() -> (w6871:bool)
                                n6433 = Or(x=w6871, y=w6870) -> (x .or. y?=w6869:bool)
                                n6434 = Wait (ms)(milliseconds to wait=u32 10) -> ()  [unwired: 1 out]
                                }
                                n6435 = One Button Dialog(message="Move to Column-2 detection zone and Press 'Start the Process' Button.") -> ()  [unwired: 1 in, 1 out]
                                }
                                frame True {
                                }
                                }
                                n6436 = local write "Volume being Injected \nin this process"(0.0 ("Volume being Injected \nin this process")) -> ()
                                n6437 = local write "Elution of Column-2"(TRUE ("Elution of Column-2")) -> ()
                                }
                                frame #20 {
                                # "If Yes, it will clean the SEC buffer from port-8 tubing else it will clean the pump valve a bit"
                                n6438 = local read "Clean the \nBuffer-C2 tubing"() -> (w6872:bool)
                                n6439 = case shown="False" w6872 {
                                frame False {
                                n6440 = stacked-sequence {
                                frame #0 {
                                n6441 = local read "VISA Refnum in\nfor Pump"() -> (w6874:refnum<visa-resource-name>)
                                n6442 = local read "Port for \nC2-Elution"() -> (w6873:string)
                                n6443 = call "PortChanger (SubVI).vi"("Port Number"=w6873, "VISA Refnum in"=w6874) -> ()  [unwired: 10 in]
                                }
                                frame #1 {
                                n6444 = local read "VISA Refnum in\nfor Pump"() -> (w6875:refnum<visa-resource-name>)
                                n6445 = call "ProcessCompletionWaiter (SubVI).vi"("VISA Refnum in"=w6875) -> ()  [unwired: 11 in]
                                }
                                frame #2 {
                                n6446 = local read "Buffer-C2 Pumping\nResolution"() -> (w6878:T2)
                                n6447 = local read "VISA Refnum in\nfor Pump"() -> (w6880:refnum<visa-resource-name>)
                                n6448 = local read "V-S"() -> (w6876:dbl)
                                n6449 = local read "Volume of Syringe"() -> (w6879:dbl)
                                n6450 = call "RPickUp(SubVI).vi"("Volume to be picked up"=w6876, "Volume of Syringe"=w6879, "Resolution of PickUP"=w6878, "PickUp Flow Rate (ul/min)"=150.0, "VISA Refnum in"=w6880) -> ()  [unwired: 6 in, 1 out]
                                }
                                frame #3 {
                                n6451 = local read "Stopper that ends \nthe main loops"() -> (w6881:bool)
                                n6452 = local read "VISA Refnum in\nfor Pump"() -> (w6882:refnum<visa-resource-name>)
                                n6453 = case shown="True" w6881 {
                                frame False {
                                }
                                frame True {
                                n6454 = local read "VISA Refnum in\nfor Pump"() -> (w6883:refnum<visa-resource-name>)
                                n6455 = call "HardStopCurrentProcess (SubVI).vi"("VISA Refnum in"=w6883) -> ()  [unwired: 11 in]
                                }
                                }
                                n6456 = call "ProcessCompletionWaiter (SubVI).vi"("VISA Refnum in"=w6882) -> ()  [unwired: 11 in]
                                }
                                frame #4 {
                                n6457 = local read "VISA Refnum in\nfor Pump"() -> (w6885:refnum<visa-resource-name>)
                                n6458 = call "PortChanger (SubVI).vi"("Port Number"="1", "VISA Refnum in"=w6885) -> ()  [unwired: 10 in]
                                }
                                frame #5 {
                                n6459 = local read "Stopper that ends \nthe main loops"() -> (w6886:bool)
                                n6460 = local read "VISA Refnum in\nfor Pump"() -> (w6887:refnum<visa-resource-name>)
                                n6461 = case shown="True" w6886 {
                                frame False {
                                }
                                frame True {
                                n6462 = local read "VISA Refnum in\nfor Pump"() -> (w6888:refnum<visa-resource-name>)
                                n6463 = call "HardStopCurrentProcess (SubVI).vi"("VISA Refnum in"=w6888) -> ()  [unwired: 11 in]
                                }
                                }
                                n6464 = call "ProcessCompletionWaiter (SubVI).vi"("VISA Refnum in"=w6887) -> ()  [unwired: 11 in]
                                }
                                frame #6 {
                                n6465 = local read "VISA Refnum in\nfor Pump"() -> (w6893:refnum<visa-resource-name>)
                                n6466 = local read "Volume of Syringe"() -> (w6890:dbl)
                                n6467 = call "GoToAbsolutePosition(SubVI).vi"("Absolute Volume Position in Syringe (in ul)"=0.0, "Volume of Syringe"=w6890, "Resolution of Pumping"=T2."Standard Pumping", "Flow Rate (ul/min)"=150.0, "VISA Refnum in"=w6893) -> ()  [unwired: 6 in, 1 out]
                                }
                                frame #7 {
                                n6468 = local read "Stopper that ends \nthe main loops"() -> (w6894:bool)
                                n6469 = local read "VISA Refnum in\nfor Pump"() -> (w6895:refnum<visa-resource-name>)
                                n6470 = case shown="True" w6894 {
                                frame False {
                                }
                                frame True {
                                n6471 = local read "VISA Refnum in\nfor Pump"() -> (w6896:refnum<visa-resource-name>)
                                n6472 = call "HardStopCurrentProcess (SubVI).vi"("VISA Refnum in"=w6896) -> ()  [unwired: 11 in]
                                }
                                }
                                n6473 = call "ProcessCompletionWaiter (SubVI).vi"("VISA Refnum in"=w6895) -> ()  [unwired: 11 in]
                                }
                                }
                                }
                                frame True {
                                n6474 = for {
                                N: 2 -> [_]
                                n6475 = stacked-sequence {
                                frame #0 {
                                n6476 = local read "VISA Refnum in\nfor Pump"() -> (w6899:refnum<visa-resource-name>)
                                n6477 = local read "Port for \nC2-Elution"() -> (w6898:string)
                                n6478 = call "PortChanger (SubVI).vi"("Port Number"=w6898, "VISA Refnum in"=w6899) -> ()  [unwired: 10 in]
                                }
                                frame #1 {
                                n6479 = local read "VISA Refnum in\nfor Pump"() -> (w6900:refnum<visa-resource-name>)
                                n6480 = call "ProcessCompletionWaiter (SubVI).vi"("VISA Refnum in"=w6900) -> ()  [unwired: 11 in]
                                }
                                frame #2 {
                                n6481 = local read "Buffer-C2 Pumping\nResolution"() -> (w6903:T2)
                                n6482 = local read "VISA Refnum in\nfor Pump"() -> (w6905:refnum<visa-resource-name>)
                                n6483 = local read "Apparent Volume\nof Syringe"() -> (w6901:dbl)
                                n6484 = local read "Volume of Syringe"() -> (w6904:dbl)
                                n6485 = call "RPickUp(SubVI).vi"("Volume to be picked up"=w6901, "Volume of Syringe"=w6904, "Resolution of PickUP"=w6903, "PickUp Flow Rate (ul/min)"=150.0, "VISA Refnum in"=w6905) -> ()  [unwired: 6 in, 1 out]
                                }
                                frame #3 {
                                n6486 = local read "Stopper that ends \nthe main loops"() -> (w6906:bool)
                                n6487 = local read "VISA Refnum in\nfor Pump"() -> (w6907:refnum<visa-resource-name>)
                                n6488 = case shown="True" w6906 {
                                frame False {
                                }
                                frame True {
                                n6489 = local read "VISA Refnum in\nfor Pump"() -> (w6908:refnum<visa-resource-name>)
                                n6490 = call "HardStopCurrentProcess (SubVI).vi"("VISA Refnum in"=w6908) -> ()  [unwired: 11 in]
                                }
                                }
                                n6491 = call "ProcessCompletionWaiter (SubVI).vi"("VISA Refnum in"=w6907) -> ()  [unwired: 11 in]
                                }
                                frame #4 {
                                n6492 = local read "VISA Refnum in\nfor Pump"() -> (w6910:refnum<visa-resource-name>)
                                n6493 = call "PortChanger (SubVI).vi"("Port Number"="1", "VISA Refnum in"=w6910) -> ()  [unwired: 10 in]
                                }
                                frame #5 {
                                n6494 = local read "Stopper that ends \nthe main loops"() -> (w6911:bool)
                                n6495 = local read "VISA Refnum in\nfor Pump"() -> (w6912:refnum<visa-resource-name>)
                                n6496 = case shown="True" w6911 {
                                frame False {
                                }
                                frame True {
                                n6497 = local read "VISA Refnum in\nfor Pump"() -> (w6913:refnum<visa-resource-name>)
                                n6498 = call "HardStopCurrentProcess (SubVI).vi"("VISA Refnum in"=w6913) -> ()  [unwired: 11 in]
                                }
                                }
                                n6499 = call "ProcessCompletionWaiter (SubVI).vi"("VISA Refnum in"=w6912) -> ()  [unwired: 11 in]
                                }
                                frame #6 {
                                n6500 = local read "VISA Refnum in\nfor Pump"() -> (w6918:refnum<visa-resource-name>)
                                n6501 = local read "Volume of Syringe"() -> (w6915:dbl)
                                n6502 = call "GoToAbsolutePosition(SubVI).vi"("Absolute Volume Position in Syringe (in ul)"=0.0, "Volume of Syringe"=w6915, "Resolution of Pumping"=T2."Standard Pumping", "Flow Rate (ul/min)"=150.0, "VISA Refnum in"=w6918) -> ()  [unwired: 6 in, 1 out]
                                }
                                frame #7 {
                                n6503 = local read "Stopper that ends \nthe main loops"() -> (w6919:bool)
                                n6504 = local read "VISA Refnum in\nfor Pump"() -> (w6920:refnum<visa-resource-name>)
                                n6505 = case shown="True" w6919 {
                                frame False {
                                }
                                frame True {
                                n6506 = local read "VISA Refnum in\nfor Pump"() -> (w6921:refnum<visa-resource-name>)
                                n6507 = call "HardStopCurrentProcess (SubVI).vi"("VISA Refnum in"=w6921) -> ()  [unwired: 11 in]
                                }
                                }
                                n6508 = call "ProcessCompletionWaiter (SubVI).vi"("VISA Refnum in"=w6920) -> ()  [unwired: 11 in]
                                }
                                }
                                }
                                }
                                }
                                }
                                frame #21 {
                                n6509 = local read "VISA Refnum in\nfor Pump"() -> (w6923:refnum<visa-resource-name>)
                                n6510 = local read "Port for \nC2-Elution"() -> (w6922:string)
                                n6511 = call "PortChanger (SubVI).vi"("Port Number"=w6922, "VISA Refnum in"=w6923) -> ()  [unwired: 10 in]
                                }
                                frame #22 {
                                n6512 = local read "VISA Refnum in\nfor Pump"() -> (w6924:refnum<visa-resource-name>)
                                n6513 = call "ProcessCompletionWaiter (SubVI).vi"("VISA Refnum in"=w6924) -> ()  [unwired: 11 in]
                                }
                                frame #23 {
                                n6514 = local read "Buffer-C2 PickUp \nFlow Rate (ul/min)"() -> (w6928:dbl)
                                n6515 = local read "Buffer-C2 Pumping\nResolution"() -> (w6927:T2)
                                n6516 = local read "VISA Refnum in\nfor Pump"() -> (w6930:refnum<visa-resource-name>)
                                n6517 = local read "Buffer-C2 Volume \nto be Pumped"() -> (w6926:dbl)
                                n6518 = local read "Volume of Syringe"() -> (w6929:dbl)
                                n6519 = call "RPickUp(SubVI).vi"("Volume to be picked up"=w6926, "Volume of Syringe"=w6929, "Resolution of PickUP"=w6927, "PickUp Flow Rate (ul/min)"=w6928, "VISA Refnum in"=w6930) -> ()  [unwired: 6 in, 1 out]
                                n6520 = local write "SEC On"(TRUE ("SEC On")) -> ()
                                }
                                frame #24 {
                                n6521 = local read "Stopper that ends \nthe main loops"() -> (w6931:bool)
                                n6522 = local read "VISA Refnum in\nfor Pump"() -> (w6932:refnum<visa-resource-name>)
                                n6523 = case shown="True" w6931 {
                                frame False {
                                }
                                frame True {
                                n6524 = local read "VISA Refnum in\nfor Pump"() -> (w6933:refnum<visa-resource-name>)
                                n6525 = call "HardStopCurrentProcess (SubVI).vi"("VISA Refnum in"=w6933) -> ()  [unwired: 11 in]
                                }
                                }
                                n6526 = call "ProcessCompletionWaiter (SubVI).vi"("VISA Refnum in"=w6932) -> ()  [unwired: 11 in]
                                }
                                frame #25 {
                                # "Reads the initial Plunger Position for computing the volume dispensed"
                                n6527 = local read "VISA Refnum in\nfor Pump"() -> (w6935:refnum<visa-resource-name>)
                                n6528 = call "AbsolutePlungerPosition (SubVI).vi"("VISA Refnum in"=w6935) -> ("Plunger Position"=w6934:i32)  [unwired: 10 in]
